vi "S71200_PLC_3.vi"(11 "Simulazione":bool) -> ()   [LabVIEW 2019]
uses:
  Uscite PLC 3.ctl
  controls/statoAO_plc_3.ctl
  StatoDO_PLC_3.ctl
  STATO PLC 3.ctl
  TypeDef_PLC_Q.ctl
  TypeDef/DEVICE NAME.ctl
  STATO PLC 1.ctl
  Uscite PLC 1.ctl
  controls/statoAO_plc_1.ctl
  StatoDO_PLC_1.ctl
  SIEMENS/S7Com_Source/S7Com_RW_CMD.ctl
  SIEMENS/S7Com_Source/S7Com_Address_Area.ctl
  SIEMENS/S7Com_Source/S7Com_Start_Add.ctl
  SIEMENS/S7Com_Source/S7Com_Transport_Size.ctl
  SIEMENS/S7Com_Source/S7Com_Function.ctl
panel:
  out "t write do":u32
  out "t write ao":u32
  out "# elements in queue":i32
  in  "millisecond multiple":u32=50
  out "write ao":errorcluster
  out "initialize":errorcluster
  in  "Tab Control":enum32{"PLC", "MERKER ", "DATABLOCK", "FGD"}(tab)
  out "STATO PLC":T1
  in  "write":bool
  in  "USCITE PLC":T2
  out "IP":string
  out "Simulazione 2":bool
  out "DESC SCRITTURE MERKER WORD (AO)":string[][](array[string])
  out "Array WORD out":dbl[](array[numeric])
  out "DESC LETTURE MERKER WORD (AI)":string[][](array[string])
  out "MW read":dbl[](array[numeric])
  out "DESC SCRITTURE MERKER BIT (DO)":string[][](array[string])
  out "stato uscite DO":bool[](array[boolean])
  out "DESC LETTURE MERKER BIT (DI)":string[][](array[string])
  out "MBit read":bool[](array[boolean])
  out "DESC SCRITTURE MERKER REAK (AO)":string[][](array[string])
  out "DESC LETTURE MERKER REAL (AI)":string[][](array[string])
  out "Array M REAL out":dbl[](array[numeric])
  out "M Real":dbl[](array[numeric]) format="%.5f"
  out "DESC SCRITTURE DB BIT (DO)":string[][](array[string])
  out "DESC LETTURE DB BIT (DI)":string[][](array[string])
  out "DESC SCRITTURE DB WORD (AO)":string[][](array[string])
  out "DESC LETTURE DB WORD (AI)":string[][](array[string])
  out "DESC LETTURE DB REAL (AI)":string[][](array[string])
  out "DESC SCRITTURE DB REAL (AO)":string[][](array[string])
  out "DB WORD":dbl[](array[numeric])
  out "DB REAL":dbl[](array[numeric]) format="%.6f"
  out "Array DB bit":bool[](array[boolean])
  out "Array DB W out":dbl[](array[numeric])
  out "Array DB REAL out":dbl[](array[numeric]) format="%#.5f"
  out "DO (DATABLOCK)":bool[](array[boolean])
  out "M BIT SCRITTURE":cluster{"M":i16, "BIT":i16[]}[](array[cluster])
  out "M BIT LETTURE":cluster{"M":i16, "BIT":i16[]}[](array[cluster])
  out "MW SCRITTURE":T5(array[cluster])
  out "MW LETTURE":T5(array[cluster])
  out "M REAL LETTURE":cluster{"MD":i16, "Descrizione":string}[](array[cluster])
  out "M REAL SCRITTURE (AO)":cluster{"MD":i16, "Descrizione":string}[](array[cluster])
  out "DBW LETTURE":T6(array[cluster])
  out "DB REAL LETTURE":T7(array[cluster])
  out "DBW SCRITTURE":T6(array[cluster])
  out "DB REAL SCRITTURE":T7(array[cluster])
  out "DB BIT LETTURE":cluster{"DB":i16, "BIT":i16[], "DBoffset":i16}[](array[cluster])
  out "DB BIT SCRITTURE":cluster{"DB":i16, "BIT":i16[], "DBoffset":i16}[](array[cluster])
  out "Message":string
  out "write do":errorcluster
  out "read":errorcluster
  out "error out":errorcluster
  out "Numeric":i32
  out "Tread ms":u32
  in  "stop":bool
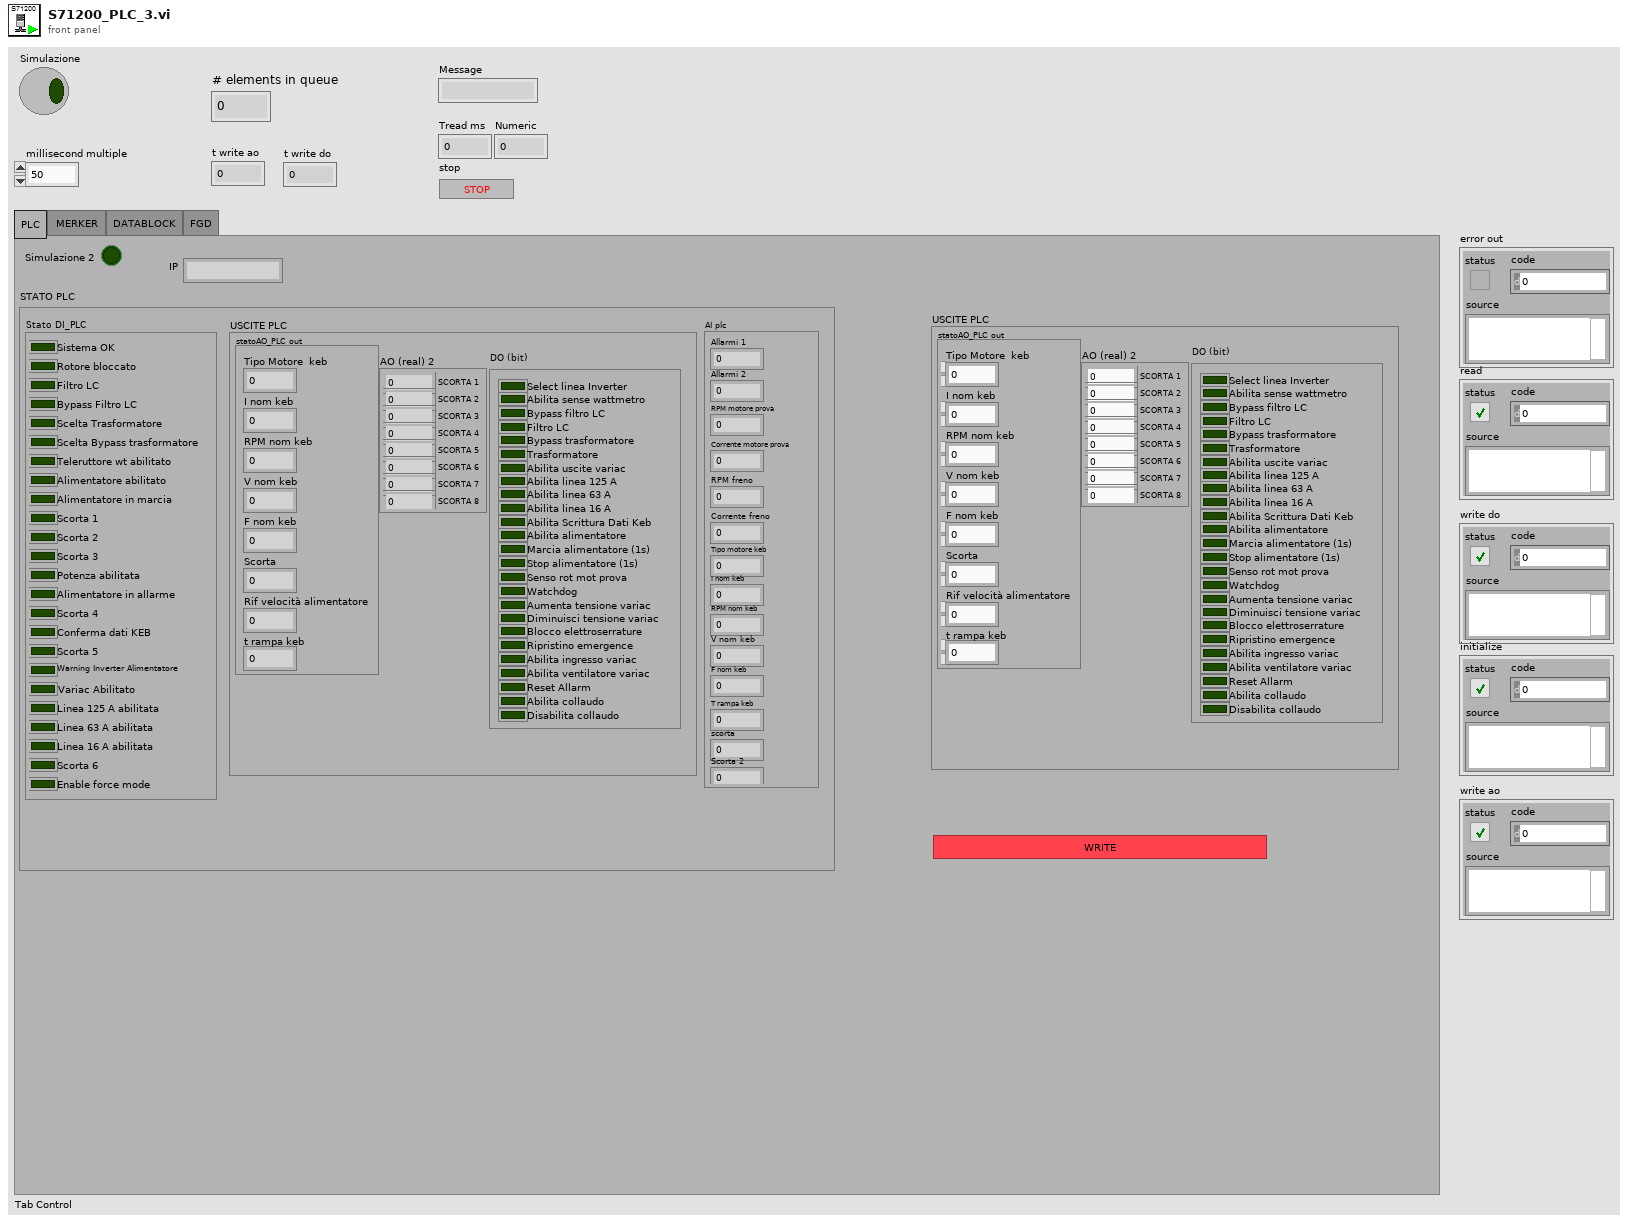
[diagram p1: front panel]
types:
  T1 = typedef "STATO PLC 3.ctl" = cluster{"USCITE PLC":T2, "Stato DI_PLC":cluster{"Sistema OK":bool, "Rotore bloccato":bool, "Filtro LC":bool, "Bypass Filtro LC":bool, "Scelta Trasformatore":bool, "Scelta Bypass trasformatore":bool, "Teleruttore wt abilitato":bool, "Alimentatore abilitato":bool, "Alimentatore in marcia":bool, "Scorta 1":bool, "Scorta 2":bool, "Scorta 3":bool, "Potenza abilitata":bool, "Alimentatore in allarme":bool, "Scorta 4":bool, "Conferma dati KEB":bool, "Scorta 5":bool, "Warning Inverter Alimentatore":bool, "Variac Abilitato":bool, "Linea 125 A abilitata":bool, "Linea 63 A abilitata":bool, "Linea 16 A abilitata":bool, "Scorta 6":bool, "Enable force mode":bool}, "AI plc":cluster{"Allarmi 1":dbl, "Allarmi 2":dbl, "RPM motore prova":dbl, "Corrente motore prova":dbl, "RPM freno":dbl, "Corrente freno":dbl, "Tipo motore keb":dbl, "I nom keb":dbl, "RPM nom keb":dbl, "V nom keb":dbl, "F nom keb":dbl, "T rampa keb":dbl, "scorta":dbl, "Scorta 2":dbl}}
  T2 = typedef "Uscite PLC 3.ctl" = cluster{"AO (real) 2":cluster{"SCORTA 1":dbl, "SCORTA 2":dbl, "SCORTA 3":dbl, "SCORTA 4":dbl, "SCORTA 5":dbl, "SCORTA 6":dbl, "SCORTA 7":dbl, "SCORTA 8":dbl}, "statoAO_PLC out":T3, "DO (bit)":T4}
  T3 = typedef "statoAO_plc_3.ctl" = cluster{"Rif velocità alimentatore":dbl, "Scorta":dbl, "Tipo Motore  keb":dbl, "I nom keb":dbl, "RPM nom keb":dbl, "V nom keb":dbl, "F nom keb":dbl, "t rampa keb":dbl}
  T4 = typedef "StatoDO_PLC_3.ctl" = cluster{"Select linea Inverter":bool, "Abilita sense wattmetro":bool, "Bypass filtro LC":bool, "Filtro LC":bool, "Bypass trasformatore":bool, "Trasformatore":bool, "Abilita uscite variac":bool, "Abilita linea 125 A":bool, "Abilita linea 63 A":bool, "Abilita linea 16 A":bool, "Abilita Scrittura Dati Keb":bool, "Abilita alimentatore":bool, "Marcia alimentatore (1s)":bool, "Stop alimentatore (1s)":bool, "Senso rot mot prova":bool, "Watchdog":bool, "Aumenta tensione variac":bool, "Diminuisci tensione variac ":bool, "Blocco elettroserrature":bool, "Ripristino emergence":bool, "Abilita ingresso variac":bool, "Abilita ventilatore variac":bool, "Reset Allarm":bool, "Scorta 1":bool, "Scorta 2":bool, "Scorta 3":bool, "Scorta 4":bool, "Scorta 5":bool, "Scorta 6":bool, "Scorta 7":bool, "Scorta 8":bool, "Scorta 9":bool, "Abilita collaudo":bool, "Disabilita collaudo ":bool, "Scorta 10":bool, "Scorta 11":bool, "Scorta 12":bool, "Scorta 13":bool, "Scorta 14":bool, "Scorta 15":bool}
  T5 = cluster{"MW":dbl, "Descrizione":string, "offset":dbl, "FS":dbl}[]
  T6 = cluster{"DB":i16, "DB offset":i16, "Descrizione":string, "offset":dbl, "FS":dbl}[]
  T7 = cluster{"DB":i16, "Descrizione":string, "DB offset":i16}[]
  T8 = typedef "TypeDef_PLC_Q.ctl" = cluster{"Message":string, "Data":variant}
  T9 = typedef "DEVICE NAME.ctl" = enum16{"WATTMETRO", "APLUS", "PLC BANCO 1", "PLC RACK", "PLC BANCO 2", "PS", "NI cDAQ", "RESISTOMAT"}
  T10 = typedef "S7Com_RW_CMD.ctl" = cluster{"Read Length":u16, "Data Block #":u16, "S7_Add_Area":T11, "Start Address":T12, "S7_Transport_Size":T13, "S7_Function":T14}
  T11 = typedef "S7Com_Address_Area.ctl" = u8
  T12 = typedef "S7Com_Start_Add.ctl" = u16
  T13 = typedef "S7Com_Transport_Size.ctl" = u8
  T14 = typedef "S7Com_Function.ctl" = u8
  T15 = cluster{cluster{string[][], cluster{"MW":dbl, "Descrizione":string, "offset":dbl, "FS":dbl}[]}, cluster{string[][], cluster{"MD":i16, "Descrizione":string}[]}, cluster{string[][], cluster{"MW":dbl, "Descrizione":string, "offset":dbl, "FS":dbl}[]}, cluster{string[][], cluster{"MD":i16, "Descrizione":string}[]}, cluster{string[][], cluster{"M":i16, "BIT":i16[]}[]}, cluster{string[][], cluster{"M":i16, "BIT":i16[]}[]}}
  T16 = cluster{cluster{string[][], cluster{"DB":i16, "DB offset":i16, "Descrizione":string, "offset":dbl, "FS":dbl}[]}, cluster{string[][], cluster{"DB":i16, "Descrizione":string, "DB offset":i16}[]}, cluster{string[][], cluster{"DB":i16, "DB offset":i16, "Descrizione":string, "offset":dbl, "FS":dbl}[]}, cluster{string[][], cluster{"DB":i16, "Descrizione":string, "DB offset":i16}[]}, cluster{string[][], cluster{"DB":i16, "BIT":i16[], "DBoffset":i16}[]}, cluster{string[][], cluster{"DB":i16, "BIT":i16[], "DBoffset":i16}[]}}
  T17 = cluster{string[][], cluster{"MW":dbl, "Descrizione":string, "offset":dbl, "FS":dbl}[]}
  T18 = cluster{string[][], cluster{"MD":i16, "Descrizione":string}[]}
  T19 = cluster{string[][], cluster{"M":i16, "BIT":i16[]}[]}
  T20 = cluster{string[][], cluster{"DB":i16, "DB offset":i16, "Descrizione":string, "offset":dbl, "FS":dbl}[]}
  T21 = cluster{string[][], cluster{"DB":i16, "Descrizione":string, "DB offset":i16}[]}
  T22 = cluster{string[][], cluster{"DB":i16, "BIT":i16[], "DBoffset":i16}[]}
  T23 = typedef "STATO PLC 1.ctl" = cluster{"USCITE PLC":T24, "Stato DI_PLC":cluster{"Sistema OK":bool, "Rotore bloccato":bool, "Scorta 1":bool, "Prova diretto inverter":bool, "Prova con filtro LC":bool, "Teleruttore WT abilitato":bool, "Alim sinus penta abilitato":bool, "Alim sinus penta in marcia":bool, "Freno abilitato":bool, "Freno in marcia":bool, "Senso rotazione freno":bool, "Potenza abilitata":bool, "Scorta 3":bool, "Scorta 4":bool, "scorta 5":bool, "scorta 6":bool}, "AI plc":cluster{"Allarmi 1":dbl, "Allarmi 2":dbl, "Scorta 1":dbl, "Scorta 2":dbl, "RPM mot prova":dbl, "I mot prova":dbl, "RPM freno":dbl, "I freno":dbl, "Scorta 3":dbl, "Scorta 4":dbl}}
  T24 = typedef "Uscite PLC 1.ctl" = cluster{"AO (real) 2":cluster{"SCORTA 1":dbl, "SCORTA 2":dbl, "SCORTA 3":dbl, "SCORTA 4":dbl, "SCORTA 5":dbl, "SCORTA 6":dbl, "SCORTA 7":dbl, "SCORTA 8":dbl}, "statoAO_PLC out":T25, "DO (bit)":T26}
  T25 = typedef "statoAO_plc_1.ctl" = cluster{"Rif Lim coppia freno [%]":dbl, "Rif rpm freno [%]":dbl, "Rif coppia freno [%]":dbl, "Rif V alimentatore [%]":dbl, "Rif F alimentatore [%]":dbl}
  T26 = typedef "StatoDO_PLC_1.ctl" = cluster{"Scelta banco 1":bool, "Set dati motore freno 2":bool, "Diretto inverter":bool, "Filtro LC":bool, "Marcia ALIM (1s)":bool, "Marcia FRENO (1s)":bool, "Stop AFE (1s)":bool, "Stop freno (1s)":bool, "Reset allarmi":bool, "Watchdog":bool, "Senso rotazione":bool, "Abilita collaudo (1s)":bool, "Disabilita collaudo (1s)":bool, "Abilitazione ALIM":bool, "Abilitazione FRENO":bool, "Teleruttore WT":bool, "Senso rot motore prova":bool, "Scorta 7":bool, "Scorta 8":bool, "Scorta 9":bool, "Scorta 10":bool, "Scorta 11":bool, "Scorta 12":bool, "Scorta 13":bool}
  T27 = cluster{"SCORTA 1":dbl, "SCORTA 2":dbl, "SCORTA 3":dbl, "SCORTA 4":dbl, "SCORTA 5":dbl, "SCORTA 6":dbl, "SCORTA 7":dbl, "SCORTA 8":dbl}
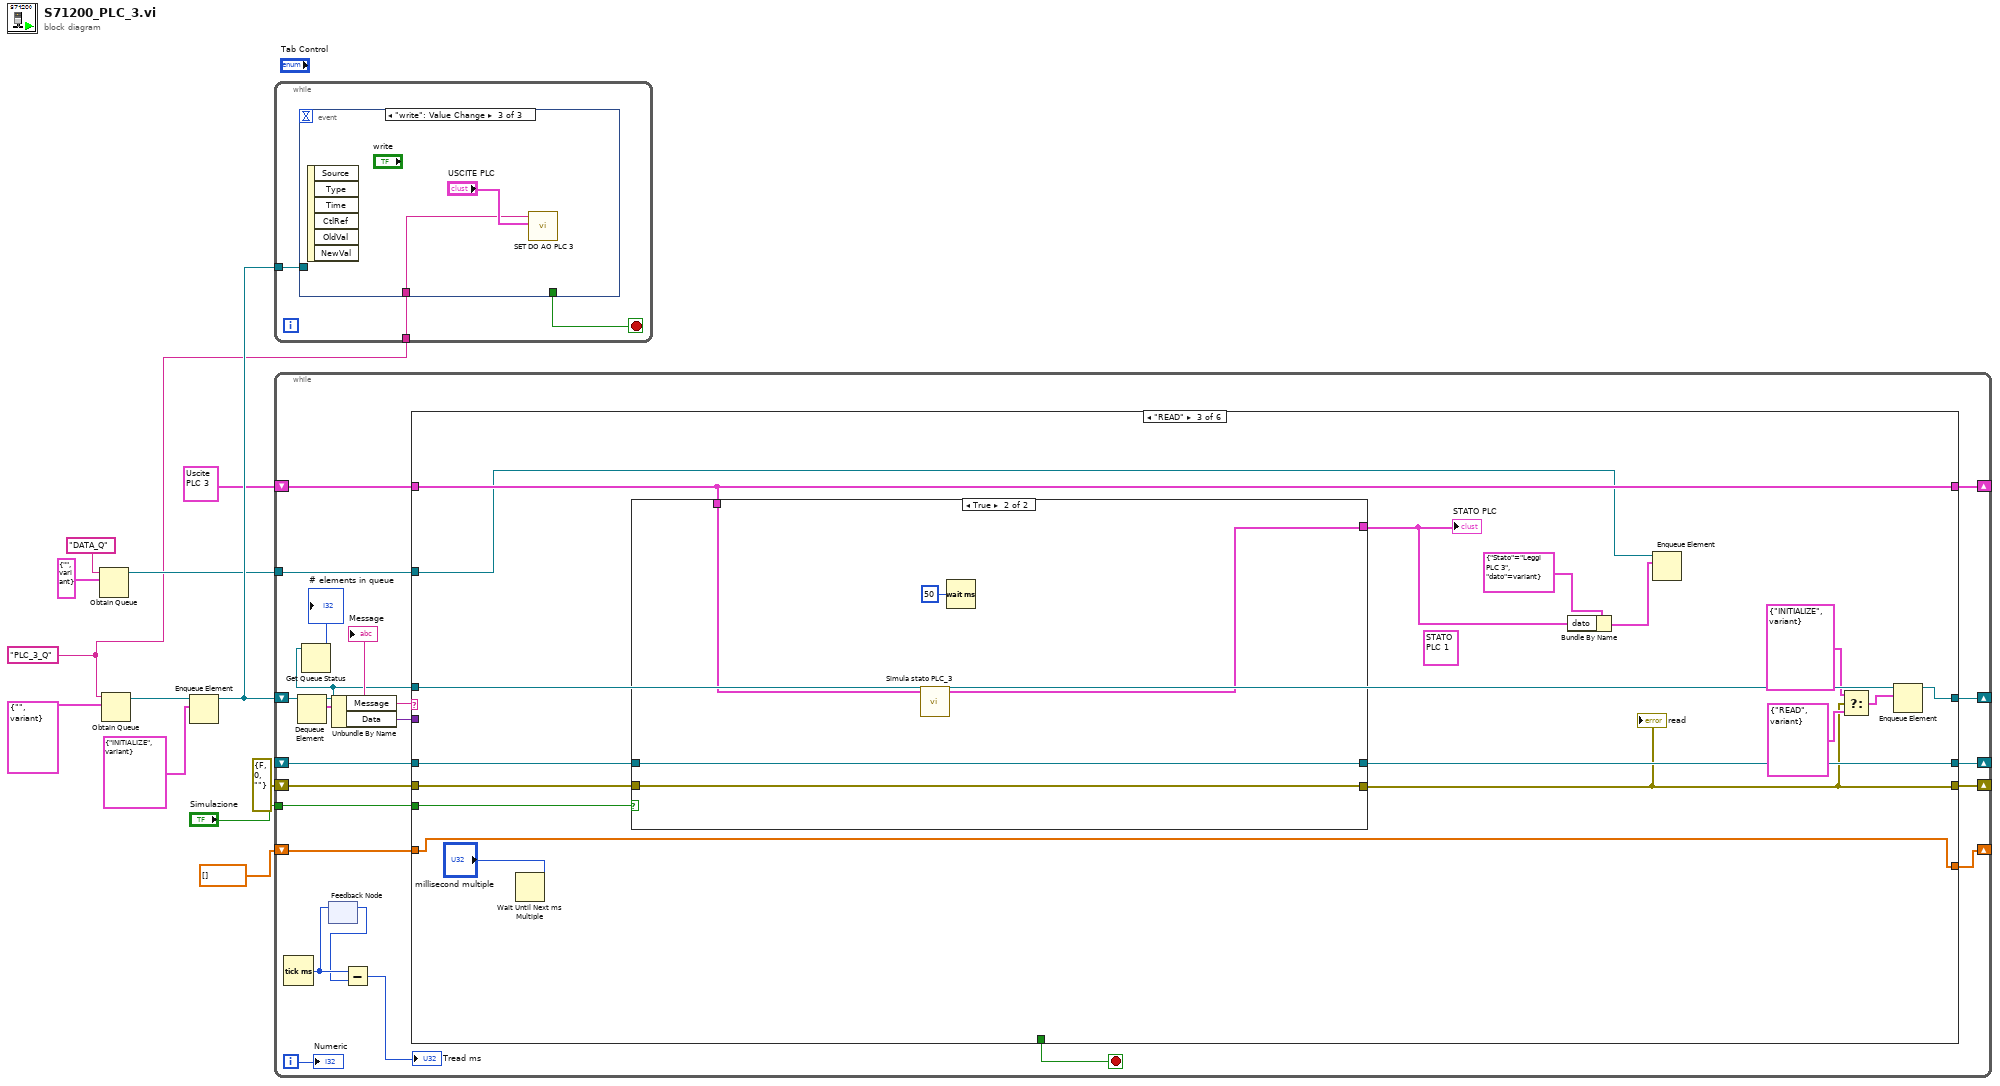
[diagram p0: block diagram]
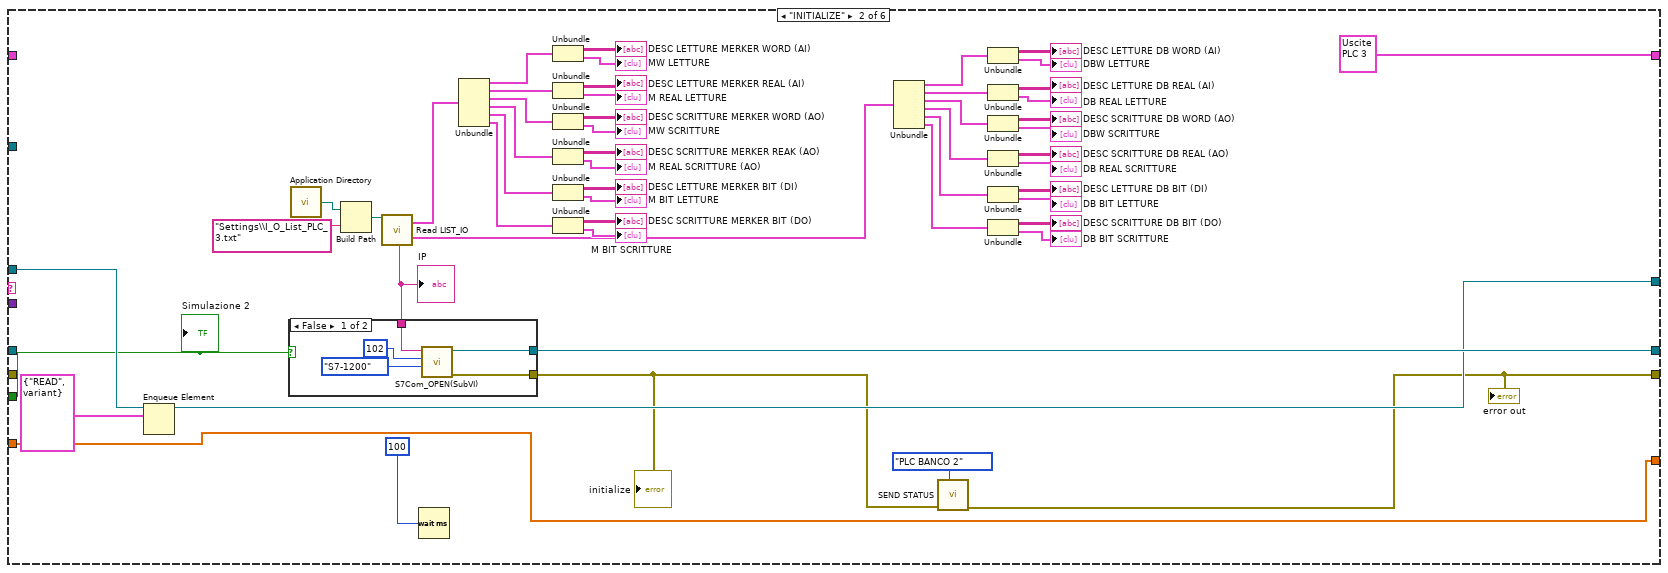
[diagram p3: hidden frame]
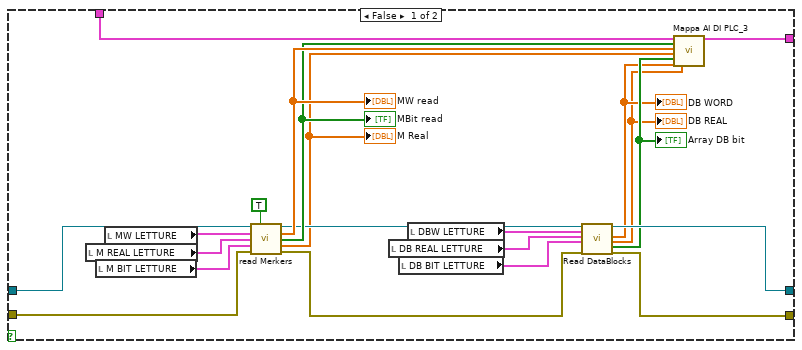
[diagram p5: hidden frame]
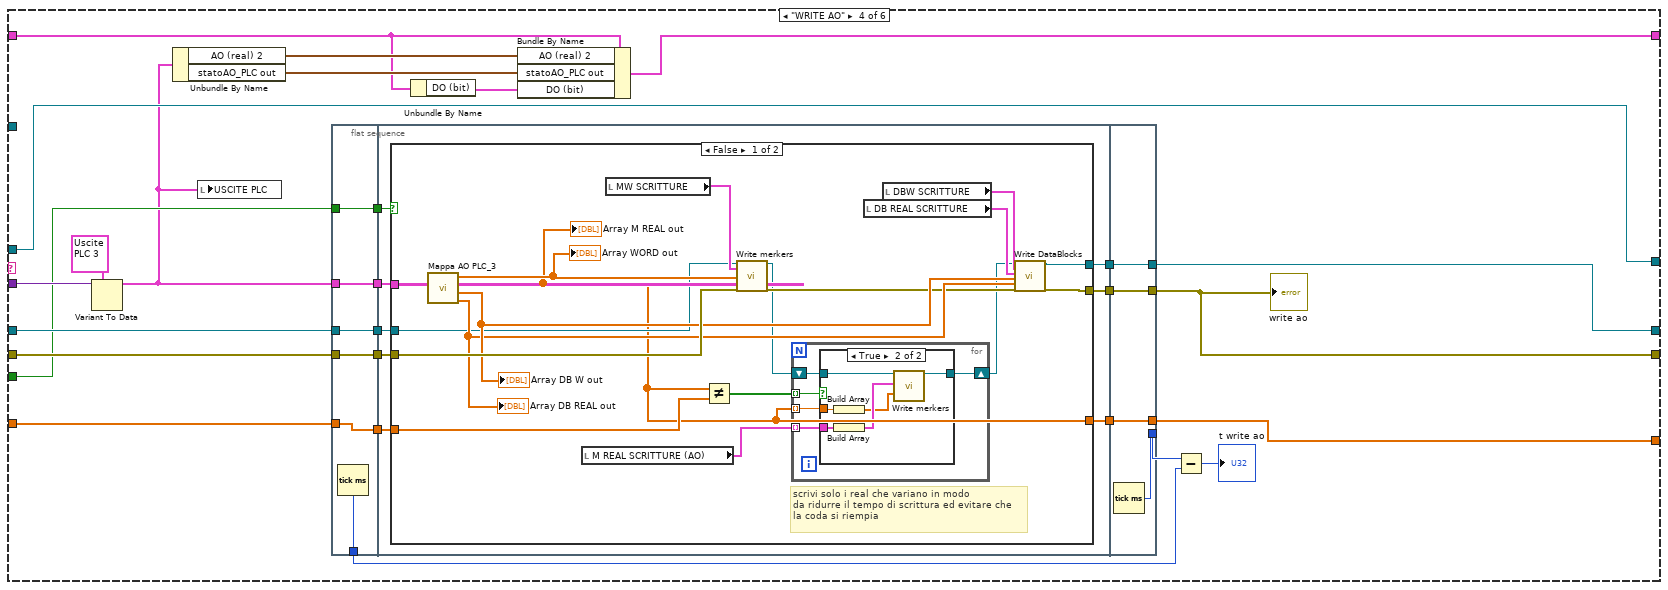
[diagram p6: hidden frame]
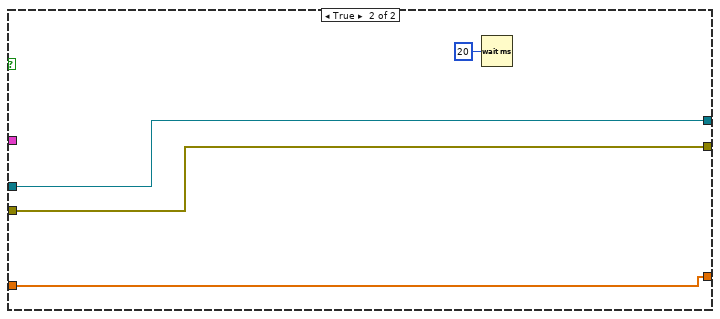
[diagram p8: hidden frame]
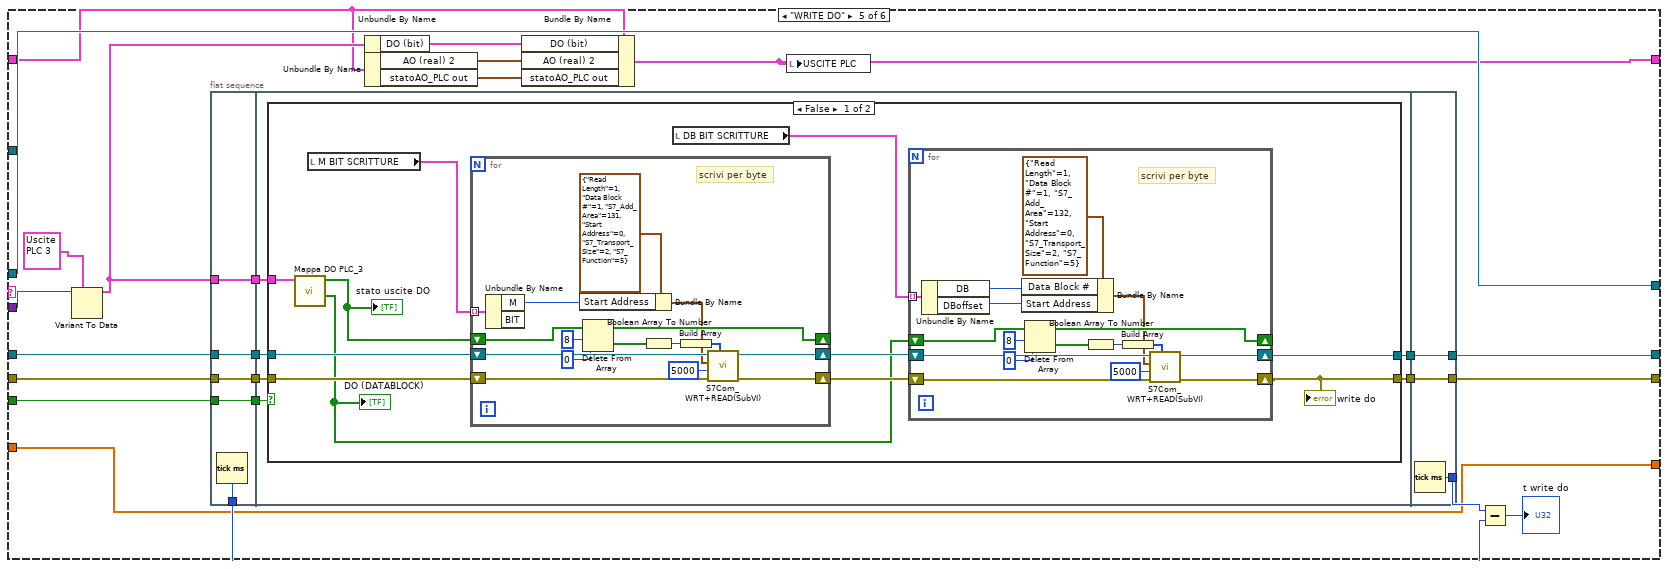
[diagram p9: hidden frame]
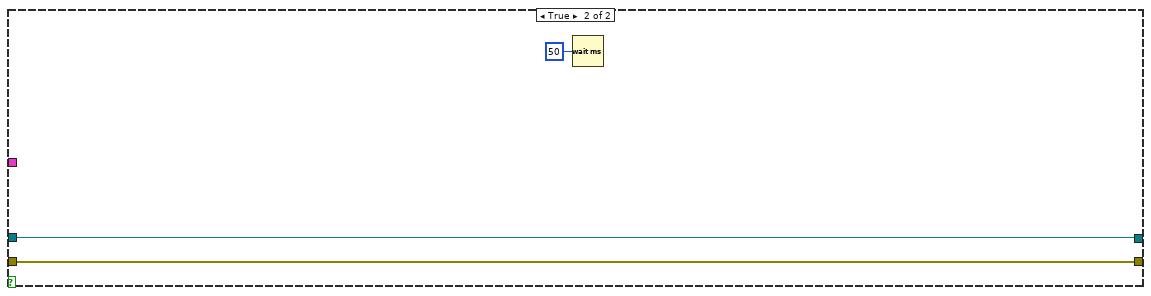
[diagram p10: hidden frame]
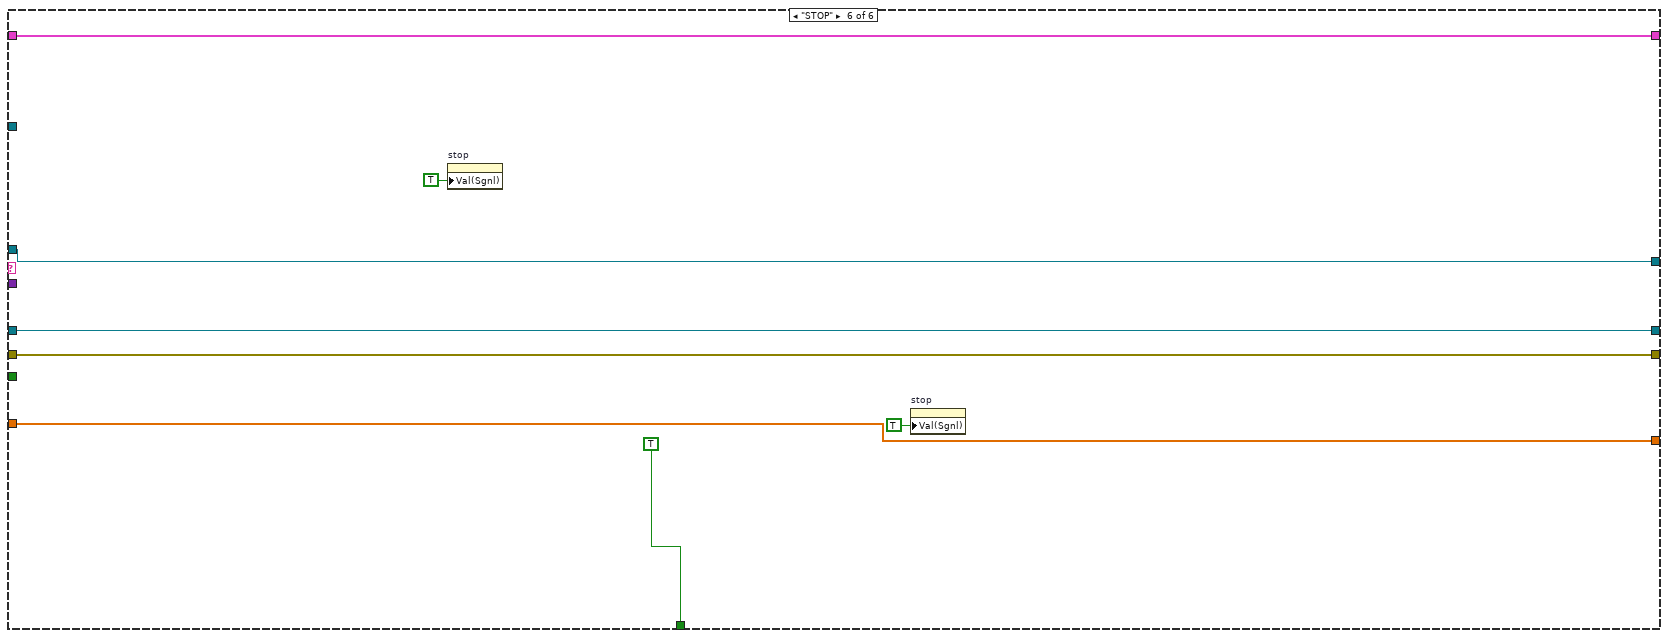
[diagram p11: hidden frame]
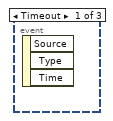
[diagram p12: hidden frame]
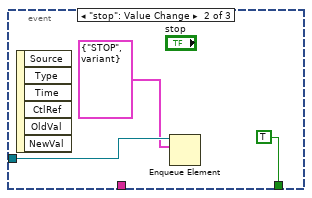
[diagram p13: hidden frame]
diagram:
  w2 = "PLC_3_Q" ("name (unnamed)")
  n1 = Obtain Queue(name (unnamed)="DATA_Q", element data type=cluster{"Stato":string, "dato":variant} {"Stato"="", "dato"=variant} ("Cluster")) -> (queue out=w4:refnum<queue>)  [unwired: 3 in, 2 out]
  n2 = Obtain Queue(name (unnamed)=w2, element data type=T8 {"Message"="", "Data"=variant}) -> (queue out=w11:refnum<queue>)  [unwired: 3 in, 2 out]
  n3 = Enqueue Element(queue=w11, element=T8 {"Message"="INITIALIZE", "Data"=variant}) -> (queue out=w10:refnum<queue>)  [unwired: 2 in, 2 out]
  n4 = while {
    tunnel: w10 -> [w14]
    tunnel: w2 -> [w13]
    stop <- w15 stop-if-true
    n5 = event shown="[2] \"write\": Value Change" {
      selector: _ -> [_ _ _]
      dyn-events: _ -> [_ _ _]
      timeout: _ -> [_ _ _]
      tunnel: [_ TRUE _] -> w15
      tunnel: w14 -> [_ w17 _]
      tunnel: w13 -> [_ _ w19]
      event Timeout {
        n6 = event-data() -> ()  [unwired: 1 in, 3 out]
      }
      event "stop": Value Change {
        n7 = event-data() -> ()  [unwired: 1 in, 6 out]
        n8 = Enqueue Element(queue=w17, element=cluster{"Message":string, "Data":variant} {"Message"="STOP", "Data"=variant}) -> ()  [unwired: 2 in, 3 out]
      }
      event "write": Value Change {
        n9 = event-data() -> ()  [unwired: 1 in, 6 out]
        n10 = call "SET DO AO PLC 3.vi"("USCITE PLC"="USCITE PLC", "Queue"=w19) -> ()  [unwired: 10 in]
      }
    }
  }
  n11 = while {
    shift-right: [w33] -> _
    shift-left: w10 -> [w39]
    shift-right: [w38] -> _
    shift-left: _ -> [w36]
    shift-right: [w37] -> _
    shift-left: errorcluster {"status"=FALSE, "code"=0, "source"=""} ("error out") -> [w35]
    shift-right: [w28] -> _
    shift-left: T2 {"AO (real) 2"={"SCORTA 1"=0.0, "SCORTA 2"=0.0, "SCORTA 3"=0.0, "SCORTA 4"=0.0, "SCORTA 5"=0.0, "SCORTA 6"=0.0, "SCORTA 7"=0.0, "SCORTA 8"=0.0}, "statoAO_PLC out"={"Rif velocità alimentatore"=0.0, "Scorta"=0.0, "Tipo Motore  keb"=0.0, "I nom keb"=0.0, "RPM nom keb"=0.0, "V nom keb"=0.0, "F nom keb"=0.0, "t rampa keb"=0.0}, "DO (bit)"={"Select linea Inverter"=FALSE, "Abilita sense wattmetro"=FALSE, "Bypass filtro LC"=FALSE, "Filtro LC"=FALSE, "Bypass trasformatore"=FALSE, "Trasformatore"=FALSE, "Abilita uscite variac"=FALSE, "Abilita linea 125 A"=FALSE, "Abilita linea 63 A"=FALSE, "Abilita linea 16 A"=FALSE, "Abilita Scrittura Dati Keb"=FALSE, "Abilita alimentatore"=FALSE, "Marcia alimentatore (1s)"=FALSE, "Stop alimentatore (1s)"=FALSE, "Senso rot mot prova"=FALSE, "Watchdog"=FALSE, "Aumenta tensione variac"=FALSE, "Diminuisci tensione variac "=FALSE, "Blocco elettroserrature"=FALSE, "Ripristino emergence"=FALSE, "Abilita ingresso variac"=FALSE, "Abilita ventilatore variac"=FALSE, "Reset Allarm"=FALSE, "Scorta 1"=FALSE, "Scorta 2"=FALSE, "Scorta 3"=FALSE, "Scorta 4"=FALSE, "Scorta 5"=FALSE, "Scorta 6"=FALSE, "Scorta 7"=FALSE, "Scorta 8"=FALSE, "Scorta 9"=FALSE, "Abilita collaudo"=FALSE, "Disabilita collaudo "=FALSE, "Scorta 10"=FALSE, "Scorta 11"=FALSE, "Scorta 12"=FALSE, "Scorta 13"=FALSE, "Scorta 14"=FALSE, "Scorta 15"=FALSE}} ("USCITE PLC 2") -> [w27]
    tunnel: "Simulazione" -> [w26]
    tunnel: w4 -> [w25]
    shift-right: [w21] -> _
    shift-left: dbl[] [] -> [w22]
    i -> [w29]
    stop <- w34 stop-if-true
    n12 = Tick Count (ms)() -> (millisecond timer value=w32:u32)
    n13 = Dequeue Element(queue=w39) -> (queue out=w24:refnum<queue>, element=w42:T8)  [unwired: 2 in, 2 out]
    n14 = Get Queue Status(queue=w24) -> (# elements in queue=→"# elements in queue":i32)  [unwired: 2 in, 7 out]
    n15 = feedback-in #1(w32) -> ()
    n16 = feedback #1() -> (w31:u32)  [unwired: 1 in]
    n17 = Unbundle By Name(w42) -> ("Message"=w41:string, "Data"=w40:variant)
    "Message" <- w41
    n18 = Subtract(x=w32, y=w31) -> (x-y=→"Tread ms":u32)
    n19 = case shown="\"READ\"" w41 {
      tunnel: w40 -> [_ _ _ w171 w248 _]
      tunnel: [w47 w100 w116 w169 w247 w319] -> w38
      tunnel: [w46 w51 w107 w170 w246 w318] -> w37
      tunnel: w36 -> [w47 _ w122 w175 w251 w319]
      tunnel: w35 -> [w46 _ w121 w174 w250 w318]
      tunnel: [_ _ _ _ _ TRUE] -> w34
      tunnel: w24 -> [w45 w95 w120 w173 w249 w317]
      tunnel: [w45 w94 w119 w173 w249 w317] -> w33
      tunnel: [w44 T2 {"AO (real) 2"={"SCORTA 1"=0.0, "SCORTA 2"=0.0, "SCORTA 3"=0.0, "SCORTA 4"=0.0, "SCORTA 5"=0.0, "SCORTA 6"=0.0, "SCORTA 7"=0.0, "SCORTA 8"=0.0}, "statoAO_PLC out"={"Rif velocità alimentatore"=0.0, "Scorta"=0.0, "Tipo Motore  keb"=0.0, "I nom keb"=0.0, "RPM nom keb"=0.0, "V nom keb"=0.0, "F nom keb"=0.0, "t rampa keb"=0.0}, "DO (bit)"={"Select linea Inverter"=FALSE, "Abilita sense wattmetro"=FALSE, "Bypass filtro LC"=FALSE, "Filtro LC"=FALSE, "Bypass trasformatore"=FALSE, "Trasformatore"=FALSE, "Abilita uscite variac"=FALSE, "Abilita linea 125 A"=FALSE, "Abilita linea 63 A"=FALSE, "Abilita linea 16 A"=FALSE, "Abilita Scrittura Dati Keb"=FALSE, "Abilita alimentatore"=FALSE, "Marcia alimentatore (1s)"=FALSE, "Stop alimentatore (1s)"=FALSE, "Senso rot mot prova"=FALSE, "Watchdog"=FALSE, "Aumenta tensione variac"=FALSE, "Diminuisci tensione variac "=FALSE, "Blocco elettroserrature"=FALSE, "Ripristino emergence"=FALSE, "Abilita ingresso variac"=FALSE, "Abilita ventilatore variac"=FALSE, "Reset Allarm"=FALSE, "Scorta 1"=FALSE, "Scorta 2"=FALSE, "Scorta 3"=FALSE, "Scorta 4"=FALSE, "Scorta 5"=FALSE, "Scorta 6"=FALSE, "Scorta 7"=FALSE, "Scorta 8"=FALSE, "Scorta 9"=FALSE, "Abilita collaudo"=FALSE, "Disabilita collaudo "=FALSE, "Scorta 10"=FALSE, "Scorta 11"=FALSE, "Scorta 12"=FALSE, "Scorta 13"=FALSE, "Scorta 14"=FALSE, "Scorta 15"=FALSE}} ("USCITE PLC 2") w117 w166 w242 w316] -> w28
      tunnel: w27 -> [w44 _ w117 w163 w241 w316]
      tunnel: w26 -> [_ w53 w115 w168 w245 _]
      tunnel: w25 -> [_ _ w111 _ _ _]
      tunnel: w22 -> [w43 w49 w106 w149 w228 w313]
      tunnel: [w43 w49 w106 w152 w228 w313] -> w21
      frame "False", Default {
      }
      frame "INITIALIZE" {
        n20 = Enqueue Element(queue=w95, element=T8 {"Message"="READ", "Data"=variant}) -> (queue out=w94:refnum<queue>)  [unwired: 2 in, 2 out]
        n21 = call <vilib>:"Application Directory.vi"() -> ("Application Directory"=w97:path)
        n22 = Build Path(base path=w97, name or relative path="Settings\\I_O_List_PLC_3.txt") -> (appended path=w96:path)
        n23 = call "Read LIST_IO.vi"("file (use dialog)"=w96) -> ("IP"=w99:string, "MERKER"=w92:T15, "DATABLOCK"=w61:T16)  [unwired: 16 in]
        "IP" <- w99
        n24 = case shown="False" w53 {
          tunnel: [w103 _] -> w100
          tunnel: [w102 _] -> w52
          tunnel: w99 -> [w101 _]
          frame False {
            n25 = call "S7Com_OPEN(SubVI).vi"("PLC type"=enum16{"S7-300", "S7-1200"}."S7-1200", "remote port"=u16 102, "remote address"=w101) -> ("error out"=w102:errorcluster, "connection ID out"=w103:refnum<k5>)  [unwired: 4 in, 3 out]
          }
          frame True {
          }
        }
        "initialize" <- w52
        n26 = Wait (ms)(milliseconds to wait=u32 100) -> ()  [unwired: 1 out]
        n27 = Unbundle(w92) -> (w91:T17, w88:T18, w87:T17, w84:T18, w83:T19, w80:T19)
        n28 = Unbundle(w91) -> (→"DESC LETTURE MERKER WORD (AI)":string[][], →"MW LETTURE":T5)
        n29 = Unbundle(w88) -> (→"DESC LETTURE MERKER REAL (AI)":string[][], →"M REAL LETTURE":cluster{"MD":i16, "Descrizione":string}[])
        n30 = Unbundle(w87) -> (→"DESC SCRITTURE MERKER WORD (AO)":string[][], →"MW SCRITTURE":T5)
        n31 = Unbundle(w84) -> (→"DESC SCRITTURE MERKER REAK (AO)":string[][], →"M REAL SCRITTURE (AO)":cluster{"MD":i16, "Descrizione":string}[])
        n32 = Unbundle(w83) -> (→"DESC LETTURE MERKER BIT (DI)":string[][], →"M BIT LETTURE":cluster{"M":i16, "BIT":i16[]}[])
        n33 = Unbundle(w80) -> (→"DESC SCRITTURE MERKER BIT (DO)":string[][], →"M BIT SCRITTURE":cluster{"M":i16, "BIT":i16[]}[])
        n34 = Unbundle(w61) -> (w62:T20, w64:T21, w65:T20, w67:T21, w68:T22, w70:T22)
        n35 = call "SEND STATUS.vi"("ELEMENT"=DEVICE_NAME."PLC BANCO 2", "error in (no error)"=w52) -> ("error out"=w51:errorcluster)  [unwired: 9 in]
        "error out" <- w51
        n36 = Unbundle(w62) -> (→"DESC LETTURE DB WORD (AI)":string[][], →"DBW LETTURE":T6)
        n37 = Unbundle(w64) -> (→"DESC LETTURE DB REAL (AI)":string[][], →"DB REAL LETTURE":T7)
        n38 = Unbundle(w65) -> (→"DESC SCRITTURE DB WORD (AO)":string[][], →"DBW SCRITTURE":T6)
        n39 = Unbundle(w67) -> (→"DESC SCRITTURE DB REAL (AO)":string[][], →"DB REAL SCRITTURE":T7)
        n40 = Unbundle(w68) -> (→"DESC LETTURE DB BIT (DI)":string[][], →"DB BIT LETTURE":cluster{"DB":i16, "BIT":i16[], "DBoffset":i16}[])
        n41 = Unbundle(w70) -> (→"DESC SCRITTURE DB BIT (DO)":string[][], →"DB BIT SCRITTURE":cluster{"DB":i16, "BIT":i16[], "DBoffset":i16}[])
        "Simulazione 2" <- w53
      }
      frame "READ" {
        (unwired) T23 {"USCITE PLC"={"AO (real) 2"={"SCORTA 1"=0.0, "SCORTA 2"=0.0, "SCORTA 3"=0.0, "SCORTA 4"=0.0, "SCORTA 5"=0.0, "SCORTA 6"=0.0, "SCORTA 7"=0.0, "SCORTA 8"=0.0}, "statoAO_PLC out"={"Rif Lim coppia freno [%]"=0.0, "Rif rpm freno [%]"=0.0, "Rif coppia freno [%]"=0.0, "Rif V alimentatore [%]"=0.0, "Rif F alimentatore [%]"=0.0}, "DO (bit)"={"Scelta banco 1"=FALSE, "Set dati motore freno 2"=FALSE, "Diretto inverter"=FALSE, "Filtro LC"=FALSE, "Marcia ALIM (1s)"=FALSE, "Marcia FRENO (1s)"=FALSE, "Stop AFE (1s)"=FALSE, "Stop freno (1s)"=FALSE, "Reset allarmi"=FALSE, "Watchdog"=FALSE, "Senso rotazione"=FALSE, "Abilita collaudo (1s)"=FALSE, "Disabilita collaudo (1s)"=FALSE, "Abilitazione ALIM"=FALSE, "Abilitazione FRENO"=FALSE, "Teleruttore WT"=FALSE, "Senso rot motore prova"=FALSE, "Scorta 7"=FALSE, "Scorta 8"=FALSE, "Scorta 9"=FALSE, "Scorta 10"=FALSE, "Scorta 11"=FALSE, "Scorta 12"=FALSE, "Scorta 13"=FALSE}}, "Stato DI_PLC"={"Sistema OK"=FALSE, "Rotore bloccato"=TRUE, "Scorta 1"=FALSE, "Prova diretto inverter"=FALSE, "Prova con filtro LC"=FALSE, "Teleruttore WT abilitato"=FALSE, "Alim sinus penta abilitato"=FALSE, "Alim sinus penta in marcia"=FALSE, "Freno abilitato"=FALSE, "Freno in marcia"=FALSE, "Senso rotazione freno"=FALSE, "Potenza abilitata"=FALSE, "Scorta 3"=FALSE, "Scorta 4"=FALSE, "scorta 5"=FALSE, "scorta 6"=FALSE}, "AI plc"={"Allarmi 1"=0.0, "Allarmi 2"=0.0, "Scorta 1"=0.0, "Scorta 2"=0.0, "RPM mot prova"=0.0, "I mot prova"=0.0, "RPM freno"=0.0, "I freno"=0.0, "Scorta 3"=0.0, "Scorta 4"=0.0}} ("STATO PLC")
        n42 = Wait Until Next ms Multiple(millisecond multiple="millisecond multiple") -> ()  [unwired: 1 out]
        n43 = case shown="True" w115 {
          tunnel: w122 -> [w142 w148]
          tunnel: w121 -> [w141 w147]
          tunnel: w117 -> [w139 w144]
          tunnel: [w138 w146] -> w108
          tunnel: [w133 w148] -> w116
          tunnel: [w131 w147] -> w107
          frame False {
            n44 = local read "M REAL LETTURE"() -> (w137:cluster{"MD":i16, "Descrizione":string}[])
            n45 = local read "M BIT LETTURE"() -> (w136:cluster{"M":i16, "BIT":i16[]}[])
            n46 = local read "MW LETTURE"() -> (w143:T5)
            n47 = call "read Merkers.vi"("TCP Network Connection in"=w142, "U16?"=TRUE, "MW LETTURE"=w143, "M REAL LETTURE"=w137, "M BIT LETTURE"=w136, "error in (no error)"=w141) -> ("TCP Network Connection out"=w134:refnum<k5>, "MW"=w140:dbl[], "Array M bit"=w135:bool[], "M Real"=w127:dbl[], "error out"=w132:errorcluster)  [unwired: 5 in]
            "MW read" <- w140
            "MBit read" <- w135
            "M Real" <- w127
            n48 = local read "DB REAL LETTURE"() -> (w129:T7)
            n49 = local read "DB BIT LETTURE"() -> (w128:cluster{"DB":i16, "BIT":i16[], "DBoffset":i16}[])
            n50 = local read "DBW LETTURE"() -> (w130:T6)
            n51 = call "Read DataBlocks.vi"("TCP Network Connection in"=w134, "DBW LETTURE"=w130, "DB REAL LETTURE"=w129, "DB BIT LETTURE"=w128, "error in (no error)"=w132) -> ("TCP Network Connection out"=w133:refnum<k5>, "DB WORD"=w125:dbl[], "DB REAL"=w124:dbl[], "Array DB bit"=w126:bool[], "error out"=w131:errorcluster)  [unwired: 10 in]
            "DB WORD" <- w125
            "DB REAL" <- w124
            "Array DB bit" <- w126
            n52 = call "Mappa AI DI PLC_3.vi"("USCITE PLC 2"=w139, "MBit read"=w135, "MW read"=w140, "M real read"=w127, "Array DB bit"=w126, "DB WORD"=w125, "DB REAL"=w124) -> ("STATO PLC"=w138:T1)  [unwired: 12 in]
          }
          frame True {
            n53 = call "Simula stato PLC_3.vi"("USCITE PLC"=w144) -> ("STATO PLC"=w146:T1)  [unwired: 10 in]
            n54 = Wait (ms)(milliseconds to wait=u32 50) -> ()  [unwired: 1 out]
          }
        }
        "read" <- w107
        "STATO PLC" <- w108
        n55 = Bundle By Name(cluster=cluster{"Stato":string, "dato":variant} {"Stato"="Leggi PLC 3", "dato"=variant} ("Cluster"), "dato"=w108) -> (w109:cluster{"Stato":string, "dato":variant})
        n56 = Enqueue Element(queue=w111, element=w109) -> ()  [unwired: 2 in, 3 out]
        n57 = Select(t=T8 {"Message"="INITIALIZE", "Data"=variant}, s=w107, f=T8 {"Message"="READ", "Data"=variant}) -> (s? t:f=w113:T8)
        n58 = Enqueue Element(queue=w120, element=w113) -> (queue out=w119:refnum<queue>)  [unwired: 2 in, 2 out]
      }
      frame "WRITE AO" {
        n59 = Variant To Data(type=T2 {"AO (real) 2"={"SCORTA 1"=0.0, "SCORTA 2"=0.0, "SCORTA 3"=0.0, "SCORTA 4"=0.0, "SCORTA 5"=0.0, "SCORTA 6"=0.0, "SCORTA 7"=0.0, "SCORTA 8"=0.0}, "statoAO_PLC out"={"Rif velocità alimentatore"=0.0, "Scorta"=0.0, "Tipo Motore  keb"=0.0, "I nom keb"=0.0, "RPM nom keb"=0.0, "V nom keb"=0.0, "F nom keb"=0.0, "t rampa keb"=0.0}, "DO (bit)"={"Select linea Inverter"=FALSE, "Abilita sense wattmetro"=FALSE, "Bypass filtro LC"=FALSE, "Filtro LC"=FALSE, "Bypass trasformatore"=FALSE, "Trasformatore"=FALSE, "Abilita uscite variac"=FALSE, "Abilita linea 125 A"=FALSE, "Abilita linea 63 A"=FALSE, "Abilita linea 16 A"=FALSE, "Abilita Scrittura Dati Keb"=FALSE, "Abilita alimentatore"=FALSE, "Marcia alimentatore (1s)"=FALSE, "Stop alimentatore (1s)"=FALSE, "Senso rot mot prova"=FALSE, "Watchdog"=FALSE, "Aumenta tensione variac"=FALSE, "Diminuisci tensione variac "=FALSE, "Blocco elettroserrature"=FALSE, "Ripristino emergence"=FALSE, "Abilita ingresso variac"=FALSE, "Abilita ventilatore variac"=FALSE, "Reset Allarm"=FALSE, "Scorta 1"=FALSE, "Scorta 2"=FALSE, "Scorta 3"=FALSE, "Scorta 4"=FALSE, "Scorta 5"=FALSE, "Scorta 6"=FALSE, "Scorta 7"=FALSE, "Scorta 8"=FALSE, "Scorta 9"=FALSE, "Abilita collaudo"=FALSE, "Disabilita collaudo "=FALSE, "Scorta 10"=FALSE, "Scorta 11"=FALSE, "Scorta 12"=FALSE, "Scorta 13"=FALSE, "Scorta 14"=FALSE, "Scorta 15"=FALSE}} ("USCITE PLC"), Variant=w171) -> (data=w167:T2)  [unwired: 1 in, 1 out]
        n60 = Unbundle By Name(w167) -> ("AO (real) 2"=w165:T27, "statoAO_PLC out"=w164:T3)
        n61 = local write "USCITE PLC"(w167) -> ()
        n62 = flat-sequence {
          tunnel: w167 -> [w178]
          tunnel: w168 -> [w179]
          tunnel: w174 -> [w180]
          tunnel: w175 -> [w181]
          tunnel: [w181] -> w161
          tunnel: [w180] -> w160
          tunnel: [w179] -> w159
          tunnel: [w178] -> w158
          tunnel: [w177] -> w154
          tunnel: [w176] -> w150
          tunnel: w149 -> [w176]
          tunnel: w161 -> [w189]
          tunnel: w160 -> [w188]
          tunnel: w159 -> [w185]
          tunnel: w158 -> [w184]
          tunnel: [w187] -> w157
          tunnel: [w186] -> w156
          tunnel: [w183] -> w151
          tunnel: w150 -> [w182]
          tunnel: [w226] -> w169
          tunnel: [w227] -> w170
          tunnel: w157 -> [w227]
          tunnel: w156 -> [w226]
          tunnel: [w225] -> w155
          tunnel: [w224] -> w152
          tunnel: w151 -> [w224]
          frame #0 {
            n63 = Tick Count (ms)() -> (millisecond timer value=w177:u32)
          }
          frame #1 {
            n64 = case shown="False" w185 {
              tunnel: w189 -> [w200 w223]
              tunnel: w188 -> [w206 w222]
              tunnel: w184 -> [w205 _]
              tunnel: [w204 w222] -> w187
              tunnel: [w190 w223] -> w186
              tunnel: [w194 w220] -> w183
              tunnel: w182 -> [w198 w220]
              frame False {
                # "scrivi solo i real che variano in modo \nda ridurre il tempo di scrittura ed evitare che\nla coda si riempia"
                n65 = call "Mappa AO PLC_3.vi"("USCITE PLC"=w205) -> ("Array DB REAL out"=w202:dbl[], "Array DB W out"=w203:dbl[], "Array M REAL out"=w194:dbl[], "Array M WORD out"=w201:dbl[])  [unwired: 7 in]
                "Array WORD out" <- w201
                "Array M REAL out" <- w194
                "Array DB W out" <- w203
                "Array DB REAL out" <- w202
                n66 = local read "M REAL SCRITTURE (AO)"() -> (w195:cluster{"MD":i16, "Descrizione":string}[])
                n67 = local read "MW SCRITTURE"() -> (w207:T5)
                n68 = Not Equal?(x=w194, y=w198) -> (x != y?=w197:bool[])
                n69 = call "Write merkers.vi"("TCP Network Connection in"=w200, "MW SCRITTURE"=w207, "AO (word)"=w201, "error in (no error)"=w206) -> ("TCP Network Connection out"=w196:refnum<k5>, "error out"=w199:errorcluster)  [unwired: 14 in]
                n70 = for {
                  tunnel: w197 -> [w212] mode=indexing
                  shift-right: [w210] -> w191
                  shift-left: w196 -> [w211]
                  tunnel: w195 -> [w209] mode=indexing
                  tunnel: w194 -> [w208] mode=indexing
                  n71 = case shown="True" w212 {
                    tunnel: w211 -> [w213 w219]
                    tunnel: [w213 w218] -> w210
                    tunnel: w209 -> [_ w217]
                    tunnel: w208 -> [_ w215]
                    frame False {
                    }
                    frame True {
                      n72 = Build Array(w215) -> (w214:dbl[])
                      n73 = Build Array(w217) -> (w216:cluster{"MD":i16, "Descrizione":string}[])
                      n74 = call "Write merkers.vi"("TCP Network Connection in"=w219, "M REAL SCRITTURE (AO)"=w216, "AO (real) in"=w214) -> ("TCP Network Connection out"=w218:refnum<k5>)  [unwired: 15 in, 1 out]
                    }
                  }
                }
                n75 = local read "DB REAL SCRITTURE"() -> (w193:T7)
                n76 = local read "DBW SCRITTURE"() -> (w192:T6)
                n77 = call "Write DataBlocks.vi"("connection ID out"=w191, "DBW SCRITTURE"=w192, "DB REAL SCRITTURE"=w193, "DB AO (word)"=w203, "DB AO (real)"=w202, "error out"=w199) -> ("connection ID out"=w190:refnum<k5>, "error out"=w204:errorcluster)  [unwired: 12 in]
              }
              frame True {
                n78 = Wait (ms)(milliseconds to wait=u32 20) -> ()  [unwired: 1 out]
              }
            }
          }
          frame #2 {
            n79 = Tick Count (ms)() -> (millisecond timer value=w225:u32)
          }
        }
        n80 = Unbundle By Name(w163) -> ("DO (bit)"=w162:T4)
        n81 = Bundle By Name(cluster=w163, "AO (real) 2"=w165, "statoAO_PLC out"=w164, "DO (bit)"=w162) -> (w166:T2)
        n82 = Subtract(x=w155, y=w154) -> (x-y=→"t write ao":u32)
        "write ao" <- w170
      }
      frame "WRITE DO" {
        n83 = Variant To Data(type=T2 {"AO (real) 2"={"SCORTA 1"=0.0, "SCORTA 2"=0.0, "SCORTA 3"=0.0, "SCORTA 4"=0.0, "SCORTA 5"=0.0, "SCORTA 6"=0.0, "SCORTA 7"=0.0, "SCORTA 8"=0.0}, "statoAO_PLC out"={"Rif velocità alimentatore"=0.0, "Scorta"=0.0, "Tipo Motore  keb"=0.0, "I nom keb"=0.0, "RPM nom keb"=0.0, "V nom keb"=0.0, "F nom keb"=0.0, "t rampa keb"=0.0}, "DO (bit)"={"Select linea Inverter"=FALSE, "Abilita sense wattmetro"=FALSE, "Bypass filtro LC"=FALSE, "Filtro LC"=FALSE, "Bypass trasformatore"=FALSE, "Trasformatore"=FALSE, "Abilita uscite variac"=FALSE, "Abilita linea 125 A"=FALSE, "Abilita linea 63 A"=FALSE, "Abilita linea 16 A"=FALSE, "Abilita Scrittura Dati Keb"=FALSE, "Abilita alimentatore"=FALSE, "Marcia alimentatore (1s)"=FALSE, "Stop alimentatore (1s)"=FALSE, "Senso rot mot prova"=FALSE, "Watchdog"=FALSE, "Aumenta tensione variac"=FALSE, "Diminuisci tensione variac "=FALSE, "Blocco elettroserrature"=FALSE, "Ripristino emergence"=FALSE, "Abilita ingresso variac"=FALSE, "Abilita ventilatore variac"=FALSE, "Reset Allarm"=FALSE, "Scorta 1"=FALSE, "Scorta 2"=FALSE, "Scorta 3"=FALSE, "Scorta 4"=FALSE, "Scorta 5"=FALSE, "Scorta 6"=FALSE, "Scorta 7"=FALSE, "Scorta 8"=FALSE, "Scorta 9"=FALSE, "Abilita collaudo"=FALSE, "Disabilita collaudo "=FALSE, "Scorta 10"=FALSE, "Scorta 11"=FALSE, "Scorta 12"=FALSE, "Scorta 13"=FALSE, "Scorta 14"=FALSE, "Scorta 15"=FALSE}} ("USCITE PLC"), Variant=w248) -> (data=w243:T2)  [unwired: 1 in, 1 out]
        n84 = flat-sequence {
          tunnel: w243 -> [w253]
          tunnel: w245 -> [w254]
          tunnel: w250 -> [w255]
          tunnel: w251 -> [w256]
          tunnel: [w256] -> w237
          tunnel: [w255] -> w236
          tunnel: [w254] -> w235
          tunnel: [w253] -> w234
          tunnel: [w252] -> w230
          tunnel: w237 -> [w262]
          tunnel: w236 -> [w261]
          tunnel: w235 -> [w258]
          tunnel: w234 -> [w257]
          tunnel: [w260] -> w233
          tunnel: [w259] -> w232
          tunnel: [w311] -> w246
          tunnel: [w312] -> w247
          tunnel: w233 -> [w312]
          tunnel: w232 -> [w311]
          tunnel: [w310] -> w231
          frame #0 {
            n85 = Tick Count (ms)() -> (millisecond timer value=w252:u32)
          }
          frame #1 {
            n86 = case shown="False" w258 {
              tunnel: w262 -> [w273 w309]
              tunnel: w261 -> [w272 w308]
              tunnel: w257 -> [w269 _]
              tunnel: [w266 w309] -> w260
              tunnel: [w265 w308] -> w259
              frame False {
                n87 = call "Mappa DO PLC_3.vi"("USCITE PLC"=w269) -> ("DO (DATABLOCK)"=w263:bool[], "DO (MERKER)"=w270:bool[])  [unwired: 9 in]
                "stato uscite DO" <- w270
                "DO (DATABLOCK)" <- w263
                n88 = local read "M BIT SCRITTURE"() -> (w271:cluster{"M":i16, "BIT":i16[]}[])
                n89 = for {
                  tunnel: w271 -> [w306] mode=indexing
                  shift-right: [w301] -> w268
                  shift-left: w272 -> [w302]
                  shift-right: [w299] -> _
                  shift-left: w270 -> [w300]
                  shift-right: [w303] -> w267
                  shift-left: w273 -> [w304]
                  # "scrivi per byte"
                  n90 = Unbundle By Name(w306) -> ("M"=w305:i16)  [unwired: 1 out]
                  n91 = Bundle By Name(cluster=T10 {"Read Length"=1, "Data Block #"=1, "S7_Add_Area"=131, "Start Address"=0, "S7_Transport_Size"=2, "S7_Function"=5} ("RW_CMD"), "Start Address"=w305) -> (w297:T10)
                  n92 = Delete From Array(array=w300, length=8, index=0) -> (deleted portion=w295:bool[], array with subset deleted=w299:bool[])
                  n93 = Boolean Array To Number(Boolean array=w295) -> (number=w293:u32)
                  n94 = Build Array(w293) -> (w296:u32[])
                  n95 = call "S7Com_WRT+READ(SubVI).vi"("Write_Data"=w296, "error in"=w302, "timeout ms (25000)"=5000, "RW_CMD"=w297, "connection ID in"=w304) -> ("error out"=w301:errorcluster, "connection ID out"=w303:refnum<k5>)  [unwired: 2 out]
                }
                n96 = local read "DB BIT SCRITTURE"() -> (w264:cluster{"DB":i16, "BIT":i16[], "DBoffset":i16}[])
                n97 = for {
                  tunnel: w264 -> [w290] mode=indexing
                  shift-right: [w285] -> w265
                  shift-left: w268 -> [w286]
                  shift-right: [w283] -> _
                  shift-left: w263 -> [w284]
                  shift-right: [w287] -> w266
                  shift-left: w267 -> [w288]
                  # "scrivi per byte"
                  n98 = Unbundle By Name(w290) -> ("DB"=w289:i16, "DBoffset"=w274:i16)
                  n99 = Bundle By Name(cluster=T10 {"Read Length"=1, "Data Block #"=1, "S7_Add_Area"=132, "Start Address"=0, "S7_Transport_Size"=2, "S7_Function"=5} ("RW_CMD"), "Data Block #"=w289, "Start Address"=w274) -> (w281:T10)
                  n100 = Delete From Array(array=w284, length=8, index=0) -> (deleted portion=w279:bool[], array with subset deleted=w283:bool[])
                  n101 = Boolean Array To Number(Boolean array=w279) -> (number=w277:u32)
                  n102 = Build Array(w277) -> (w280:u32[])
                  n103 = call "S7Com_WRT+READ(SubVI).vi"("Write_Data"=w280, "error in"=w286, "timeout ms (25000)"=5000, "RW_CMD"=w281, "connection ID in"=w288) -> ("error out"=w285:errorcluster, "connection ID out"=w287:refnum<k5>)  [unwired: 2 out]
                }
                "write do" <- w265
              }
              frame True {
                n104 = Wait (ms)(milliseconds to wait=u32 50) -> ()  [unwired: 1 out]
              }
            }
          }
          frame #2 {
            n105 = Tick Count (ms)() -> (millisecond timer value=w310:u32)
          }
        }
        n106 = Unbundle By Name(w243) -> ("DO (bit)"=w244:T4)
        n107 = Unbundle By Name(w241) -> ("AO (real) 2"=w239:T27, "statoAO_PLC out"=w240:T3)
        n108 = Bundle By Name(cluster=w241, "DO (bit)"=w244, "AO (real) 2"=w239, "statoAO_PLC out"=w240) -> (w242:T2)
        n109 = local write "USCITE PLC"(w242) -> ()
        n110 = Subtract(x=w231, y=w230) -> (x-y=→"t write do":u32)
      }
      frame "STOP" {
        n111 = property on="stop" class="Bool (strict)"("Val(Sgnl)"=TRUE ("Value (Signaling)")) -> ()  [unwired: 2 in, 2 out]
        n112 = property on="stop" class="Bool (strict)"("Val(Sgnl)"=TRUE ("Value (Signaling)")) -> ()  [unwired: 2 in, 2 out]
      }
    }
    "Numeric" <- w29
  }
